vi "New Targets Info.vi"(1 "theta":dbl, 2 "z":dbl, 3 "y":dbl, 4 "x":dbl format="%#_13g") -> (0 "Targets Info":T1)   [LabVIEW 2016]
uses:
  Targets Info.ctl
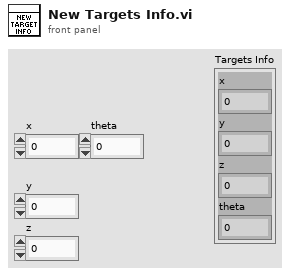
[diagram p1: front panel]
types:
  T1 = typedef "Targets Info.ctl" = cluster{"x":dbl, "y":dbl, "z":dbl, "theta":dbl}
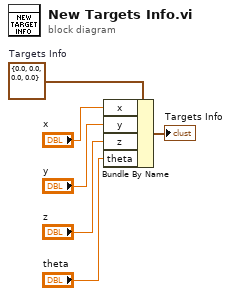
[diagram p0: block diagram]
diagram:
  w3 = T1 {"x"=0.0, "y"=0.0, "z"=0.0, "theta"=0.0}  # Targets Info
  n1 = Bundle By Name(cluster=w3, "x"="x", "y"="y", "z"="z", "theta"="theta") -> (→"Targets Info":T1)
